vi "Factory.vi"(7 "Initial Value":variant, 8 "error in (no error)":errorcluster, 9 "Ctl Refnum":refnum<vi>, 10 "Type":T1, 11 "Name":string) -> (0 "error out":errorcluster, 3 "Control out":refnum<class "Control.lvclass">)   [LabVIEW 2020, in "Aether Engine.lvlib" / "Control.lvclass"]
uses:
  Control.lvclass
  Control Data Type.ctl
  Double Control/Double Control.lvclass
  C:/dev/lv 2020/lv-aether/Aether Engine/Control/Control.lvclass
  Bool Control/Bool Control.lvclass
  Chart Control/Chart Control.lvclass
  Control.lvclass/Control.ctl
  Aether Engine.lvlib
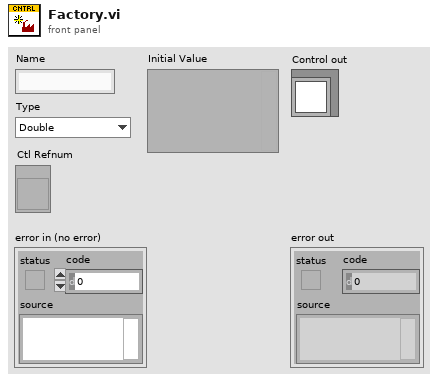
[diagram p1: front panel]
types:
  T1 = typedef "Aether Engine.lvlib/Control Data Type.ctl" = enum16{"Double", "Bool", "Chart"}
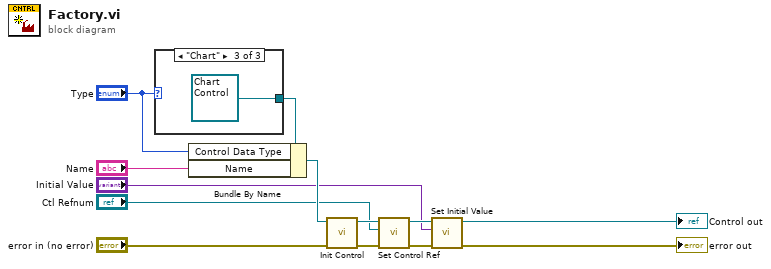
[diagram p0: block diagram]
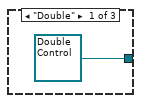
[diagram p2: hidden frame]
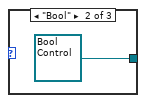
[diagram p3: hidden frame]
diagram:
  n1 = case shown="\"Chart\"" "Type" {
    tunnel: [refnum<class "Double Control.lvclass"> refnum ("Aether Engine.lvlib:Double Control.lvclass") refnum<class "Bool Control.lvclass"> refnum ("Aether Engine.lvlib:Bool Control.lvclass") refnum<class "Chart Control.lvclass"> refnum ("Aether Engine.lvlib:Chart Control.lvclass")] -> w12
    frame "Double" {
    }
    frame "Bool" {
    }
    frame "Chart" {
    }
  }
  n2 = Bundle By Name(cluster=w12, "Control Data Type"="Type", "Name"="Name") -> (w9:refnum<class "Control.lvclass">)
  n3 = call-dynamic "Init Control.vi"("error in (no error)"="error in (no error)", "Control in"=w9) -> ("error out"=w8:errorcluster, "Control out"=w7:refnum<class "Control.lvclass">)  [unwired: 8 in]
  n4 = call-dynamic "Set Control Ref.vi"("error in (no error)"=w8, "Ctl Refnum"="Ctl Refnum", "Control in"=w7) -> ("error out"=w5:errorcluster, "Control out"=w3:refnum<class "Control.lvclass">)  [unwired: 7 in]
  n5 = call-dynamic "Set Initial Value.vi"("error in (no error)"=w5, "Default Value"="Initial Value", "Control in"=w3) -> ("error out"=→"error out":errorcluster, "Control out"=→"Control out":refnum<class "Control.lvclass">)  [unwired: 7 in]
